vi "2 maximize_this.vi"(1 "Phi":dbl, 3 "Theta":dbl) -> (0 "Value":dbl)   [LabVIEW 2011]
doc: "A mathematical function derived from what we know about the boat's path. Maximizing this function is part of minimizing travel time."
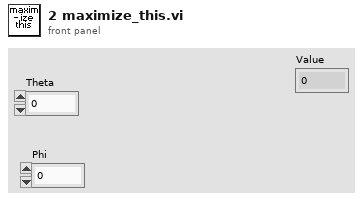
[diagram p1: front panel]
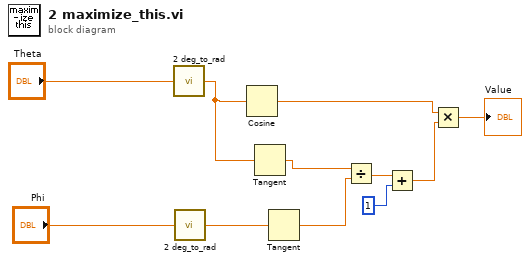
[diagram p0: block diagram]
diagram:
  n1 = call "2 deg_to_rad.vi"("Degrees"="Theta") -> ("Radians"=w4:dbl)
  n2 = call "2 deg_to_rad.vi"("Degrees"="Phi") -> ("Radians"=w3:dbl)
  n3 = Cosine(x=w4) -> (cos(x)=w6:dbl)
  n4 = Tangent(1:w4) -> (0:w11:dbl)
  n5 = Tangent(1:w3) -> (0:w10:dbl)
  n6 = Divide(x=w11, y=w10) -> (x/y=w9:dbl)
  n7 = Add(x=w9, y=1) -> (x+y=w7:dbl)
  n8 = Multiply(x=w6, y=w7) -> (x*y=→"Value":dbl)
